vi "Example Graph - Sensor Data Callback.vi"(4 "SensorDate":refnum<user-event>, 5 "Event Data":T1, 6 "Control Ref":refnum<k24>, 7 "Event Common Data":T2) -> ()   [LabVIEW 2013]
uses:
  C:/tf/play/labview/Tinkerforge.dll
  Tinkerforge.dll
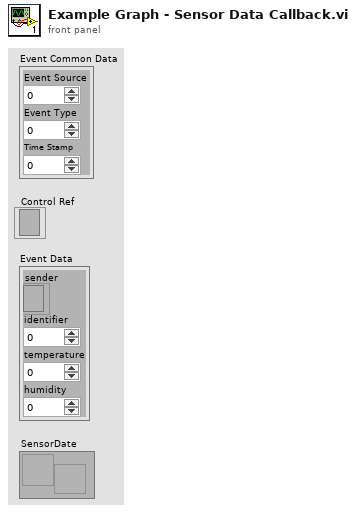
[diagram p1: front panel]
types:
  T1 = cluster{"sender":refnum<k24>, "identifier":u8, "temperature":i16, "humidity":u8}
  T2 = cluster{"Event Source":i32, "Event Type":u32, "Time Stamp":u32}
  T3 = cluster{"humidity":u8, "identifier":u8, "temperature":i16}
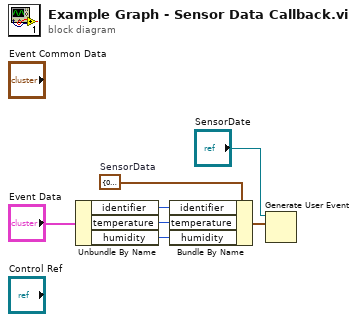
[diagram p0: block diagram]
diagram:
  w6 = T3 {"humidity"=0, "identifier"=0, "temperature"=0}  # SensorData
  n1 = Unbundle By Name("Event Data") -> ("identifier"=w5:u8, "temperature"=w4:i16, "humidity"=w3:u8)
  n2 = Bundle By Name(cluster=w6, "identifier"=w5, "temperature"=w4, "humidity"=w3) -> (w2:T3)
  n3 = Generate User Event(user event="SensorDate", event data cluster=w2) -> ()  [unwired: 2 in, 2 out]
